vi "Read_CSV_Files_9234x2.vi"() -> ()   [LabVIEW 2022 SP3]
uses:
  <vilib>/express/express analysis/Spectral/Block/exnSpectralBlock spectral measurements peak poly.vi
  <vilib>/express/express analysis/Spectral/Block/exnSpectralBlock spectral measurements peak DDT.vi
  <vilib>/ErrorRing/Error Ring.xnode
  <vilib>/express/express analysis/Spectral/XNode/ExpressSpectralMeasurementsBlockNode.xnode
panel:
  in  "Rechose":bool
  in  "Rescan":bool
  in  "Data Connect":bool
  in  "FFT export":bool
  out "選擇/總資料":string
  in  "Filenames":i32(listbox)
  out "error out":errorcluster
  out "Timedomain":dynamicdata(graph)
  out "FFT":dynamicdata(graph)
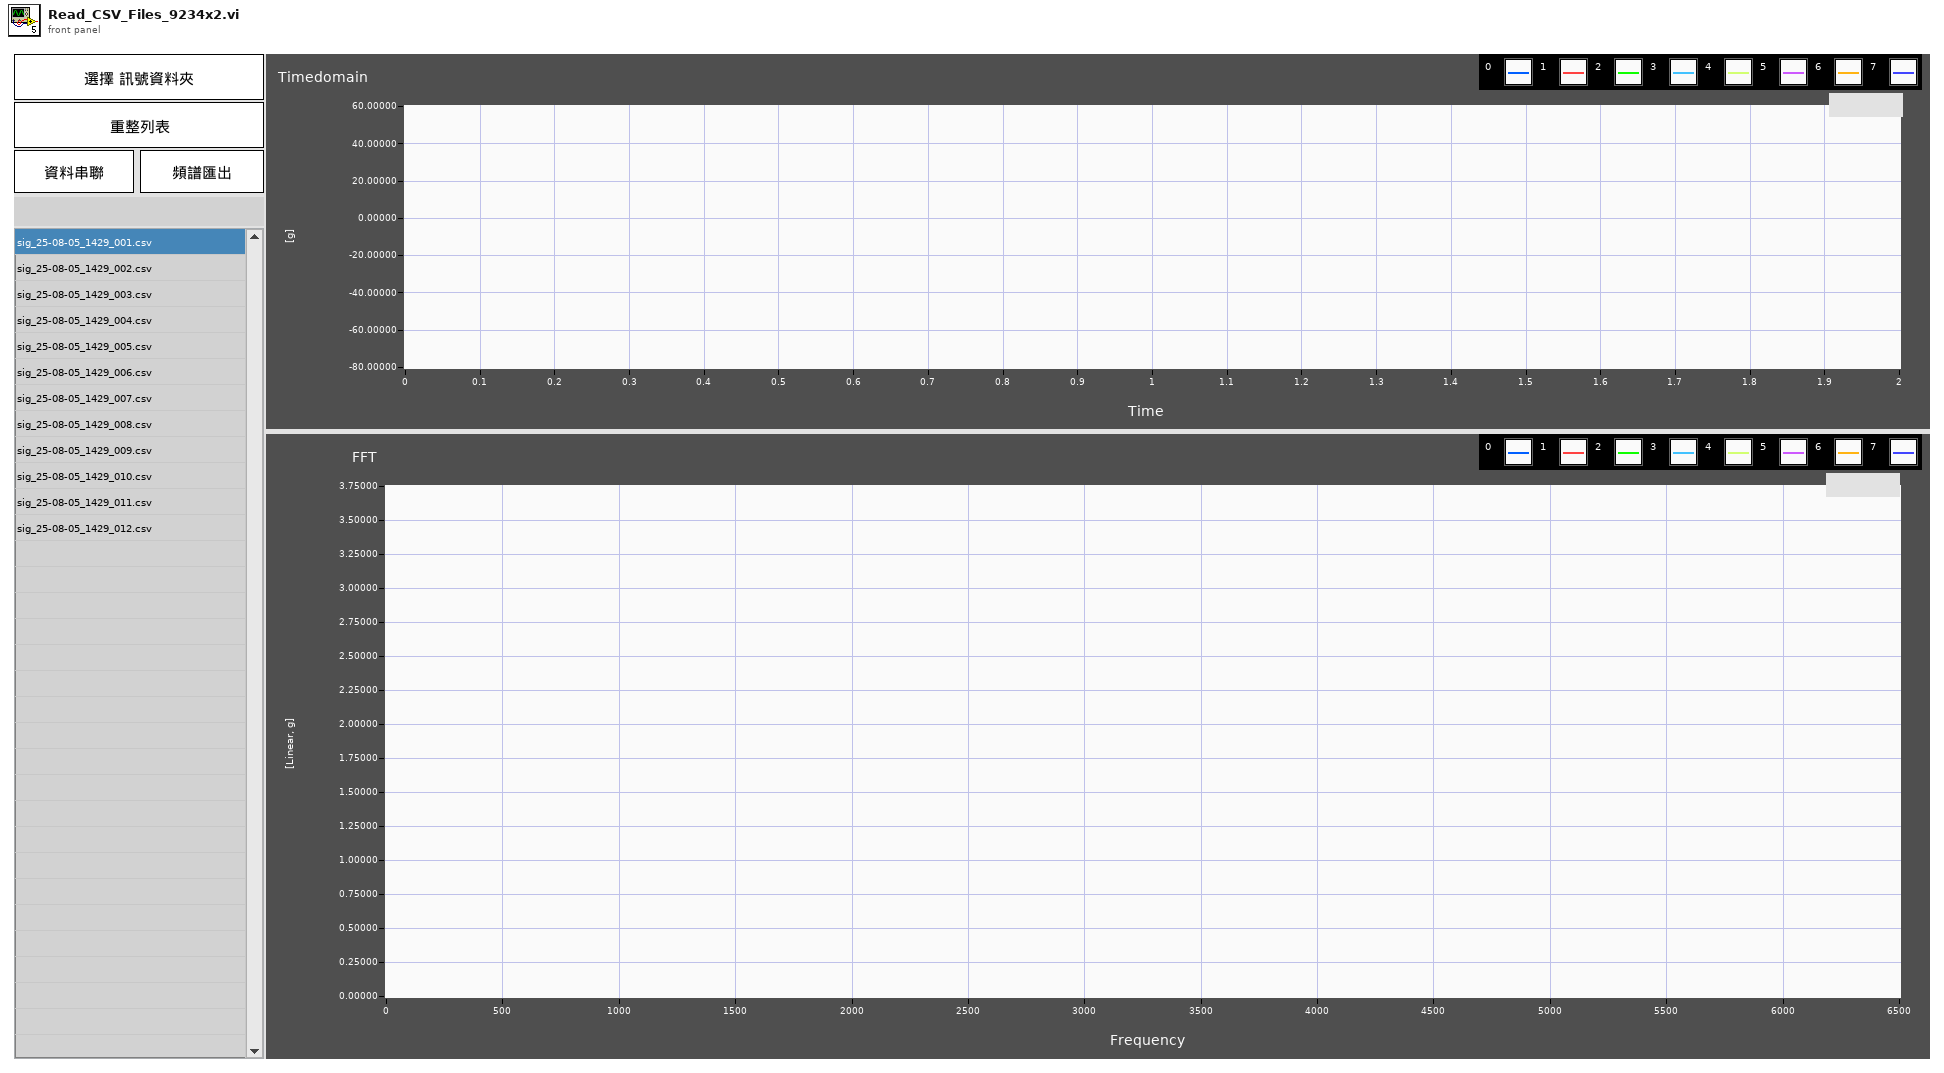
[diagram p1: front panel]
types:
  T1 = cluster{"averaging mode":u16, "weighting mode":u16, "number of averages":u32}
  T2 = cluster{"dB On (F)":bool, "unwrap phase (F)":bool, "convert to degree (F)":bool}
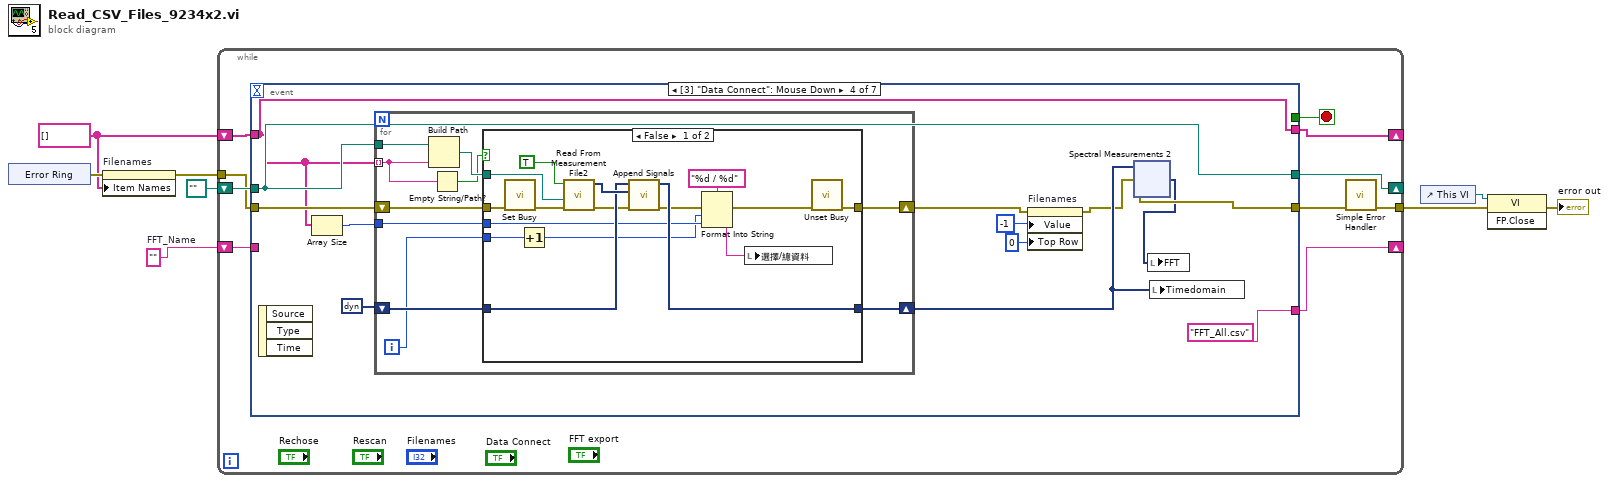
[diagram p0: block diagram]
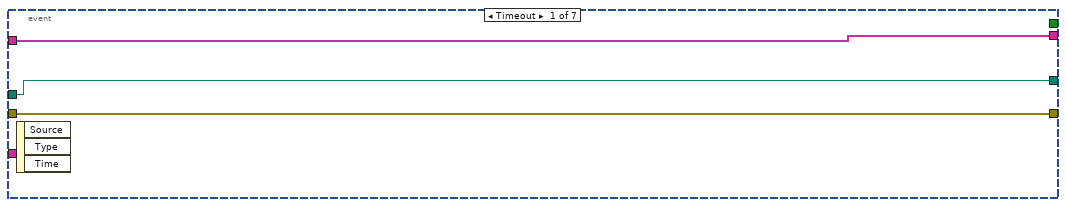
[diagram p2: hidden frame]
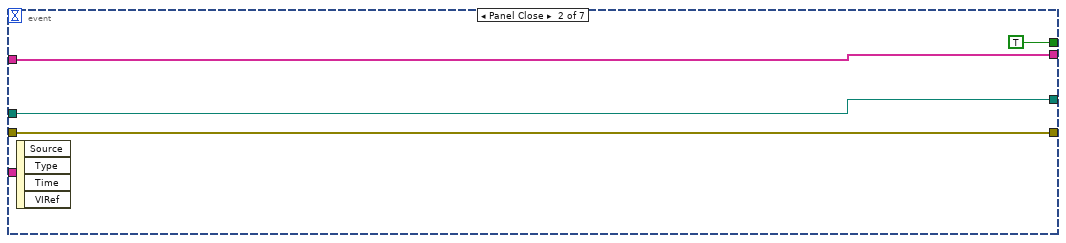
[diagram p3: hidden frame]
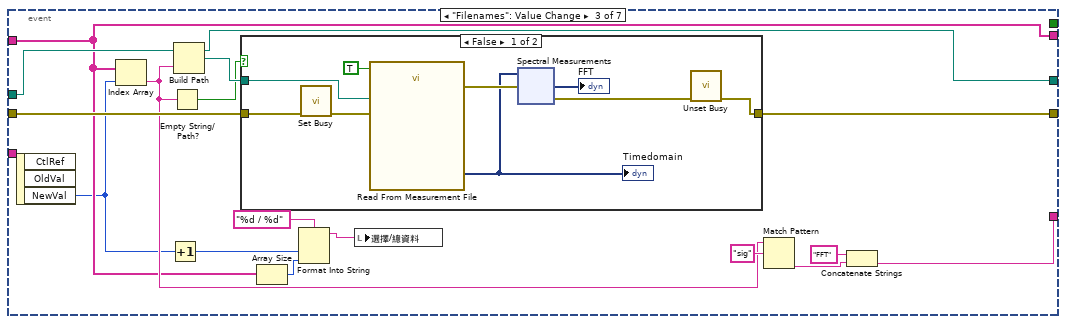
[diagram p4: hidden frame]
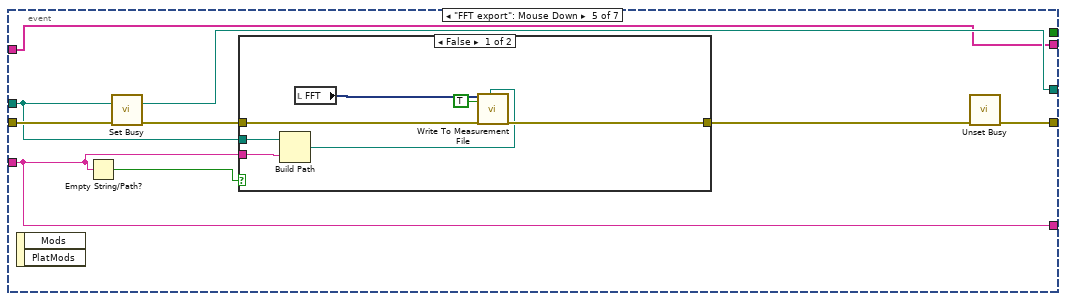
[diagram p7: hidden frame]
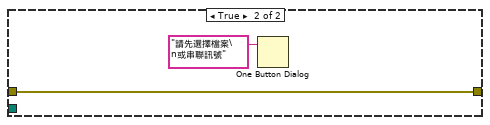
[diagram p8: hidden frame]
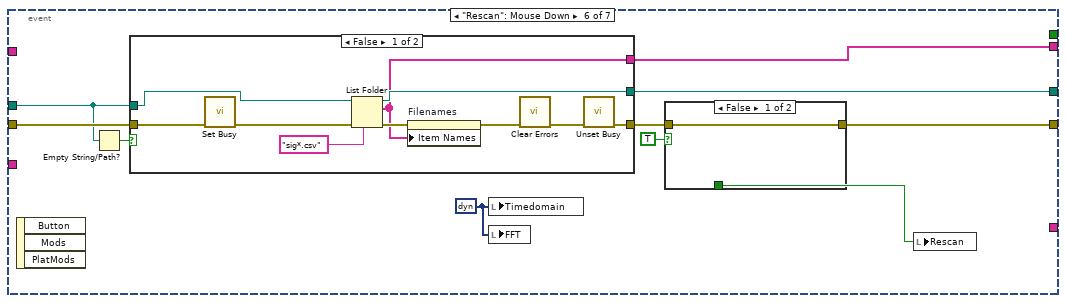
[diagram p9: hidden frame]
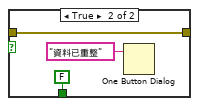
[diagram p10: hidden frame]
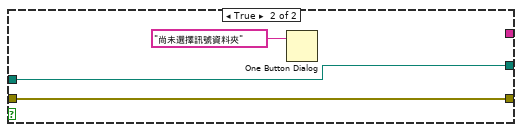
[diagram p11: hidden frame]
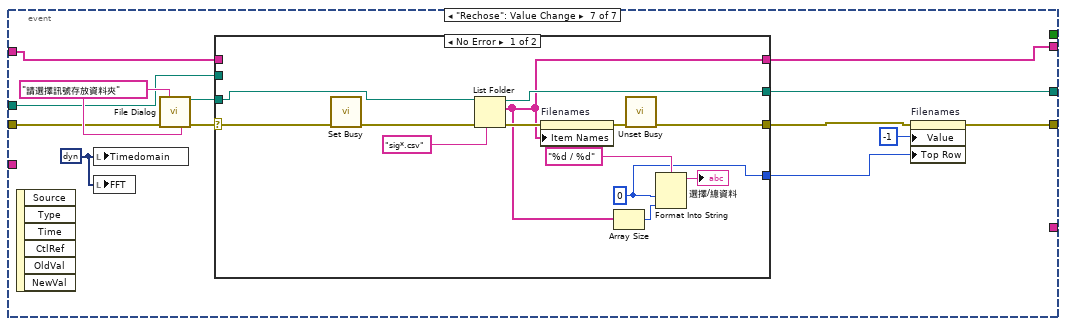
[diagram p12: hidden frame]
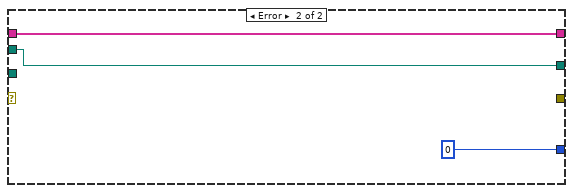
[diagram p13: hidden frame]
diagram:
  w1 = ""  # FFT_Name
  w2 = string[] [] ("filenames")
  n1 = xnode "Error Ring"() -> ("error out"=w4:errorcluster)
  n2 = property on="Filenames" class="LstBox (strict)"(error in=w4, "Item Names"=w2) -> (error out=w3:errorcluster)  [unwired: 1 in, 1 out]
  n3 = while {
    tunnel: [w14] -> w6
    shift-right: [w12] -> _
    shift-left: w2 -> [w16]
    shift-right: [w13] -> _
    shift-left: path "" ("path out") -> [w17]
    tunnel: w3 -> [w11]
    shift-right: [w10] -> _
    shift-left: w1 -> [w9]
    stop <- w18 stop-if-true
    n4 = event shown="[3] \"Data Connect\": Mouse Down" {
      selector: _ -> [_ _ _ _ _ _ _]
      dyn-events: _ -> [_ _ _ _ _ _ _]
      timeout: _ -> [_ _ _ _ _ _ _]
      tunnel: [w21 w24 w41 w72 w118 w132 w159] -> w15
      tunnel: [_ TRUE _ _ _ _ _] -> w18
      tunnel: w17 -> [w20 w23 w37 w73 w114 w136 w165]
      tunnel: w16 -> [w19 w22 w29 w67 w113 _ w164]
      tunnel: [w20 w23 w37 w73 w114 w139 w166] -> w13
      tunnel: [w19 w22 w29 w67 w113 w138 w167] -> w12
      tunnel: w11 -> [w21 w24 w38 w74 w120 w137 w162]
      tunnel: [_ _ w32 "FFT_All.csv" w115 _ _] -> w10
      tunnel: w9 -> [_ _ _ _ w115 _ _]
      event Timeout {
        n5 = event-data() -> ()  [unwired: 1 in, 3 out]
      }
      event Panel Close {
        n6 = event-data() -> ()  [unwired: 1 in, 4 out]
      }
      event "Filenames": Value Change {
        n7 = event-data() -> ("NewVal"=w28:i32)  [unwired: 1 in, 2 out]
        n8 = Index Array(array=w29, index=w28) -> (element=w33:string)
        n9 = Increment(x=w28) -> (x+1=w26:i32)
        n10 = Empty String/Path?(string/path=w33) -> (empty?=w39:bool)
        n11 = Build Path(base path=w37, name or relative path=w33) -> (appended path=w40:path)
        n12 = case shown="False" w39 {
          tunnel: [w47 w61] -> w41
          tunnel: w40 -> [w50 _]
          tunnel: w38 -> [w46 w61]
          frame False {
            n13 = call <vilib>:"Set Busy.vi"("error in (no error)"=w46) -> ("error out"=w48:errorcluster)  [unwired: 9 in, 1 out]
            n14 = call "Read From Measurement File"("error in (no error)"=w48, "Filename"=w50, "Reset"=TRUE) -> ("error out"=w45:errorcluster, "Signals"=w42:dynamicdata)  [unwired: 3 in, 4 out]
            "Timedomain" <- w42
            n15 = xnode ("Spectral Measurements")("Signals"=w42, "error in (no error)"=w45) -> ("FFT - (Peak)"=→"FFT":dynamicdata, "error out"=w44:errorcluster)  [unwired: 1 out]
            n16 = call <vilib>:"Unset Busy.vi"("error in (no error)"=w44) -> ("error out"=w47:errorcluster)  [unwired: 10 in]
          }
          frame True {
          }
        }
        n17 = Array Size(array=w29) -> (size(s)=w30:i32)
        n18 = Format Into String(format string="%d / %d", w26, w30) -> (resulting string=w27:string)  [unwired: 2 in, 1 out]
        n19 = local write "選擇/總資料"(w27) -> ()
        n20 = Match Pattern(string=w33, regular expression="sig") -> (after substring=w35:string)  [unwired: 1 in, 3 out]
        n21 = Concatenate Strings("FFT" ("string"), w35) -> (w32:string)
      }
      event "Data Connect": Mouse Down {
        n22 = event-data() -> ()  [unwired: 1 in, 3 out]
        n23 = Array Size(array=w67) -> (size(s)=w68:i32)
        n24 = for {
          tunnel: w73 -> [w89]
          tunnel: w67 -> [w92] mode=indexing
          shift-right: [w94] -> w65
          shift-left: w74 -> [w90]
          shift-right: [w87] -> w71
          shift-left: dynamicdata [] ("Signals") -> [w88]
          tunnel: w68 -> [w86]
          i -> [w85]
          n25 = Build Path(base path=w89, name or relative path=w92) -> (appended path=w93:path)
          n26 = Empty String/Path?(string/path=w92) -> (empty?=w91:bool)
          n27 = case shown="False" w91 {
            tunnel: [w107 w112] -> w94
            tunnel: w93 -> [w110 _]
            tunnel: w90 -> [w106 w112]
            tunnel: w88 -> [w104 w111]
            tunnel: [w103 w111] -> w87
            tunnel: w86 -> [w97 _]
            tunnel: w85 -> [w96 _]
            frame False {
              n28 = call <vilib>:"Set Busy.vi"("error in (no error)"=w106) -> ("error out"=w108:errorcluster)  [unwired: 9 in, 1 out]
              n29 = Increment(x=w96) -> (x+1=w95:i32)
              n30 = call "Read From Measurement File2"("error in (no error)"=w108, "Filename"=w110, "Reset"=TRUE) -> ("error out"=w102:errorcluster, "Signals"=w105:dynamicdata)  [unwired: 3 in, 4 out]
              n31 = call "Append Signals"("error in (no error)"=w102, "Input Signal B"=w105, "Input Signal A"=w104) -> ("error out"=w99:errorcluster, "Appended Signals"=w103:dynamicdata)  [unwired: 7 in]
              n32 = Format Into String(format string="%d / %d", error in=w99, w95, w97) -> (resulting string=w101:string, error out=w98:errorcluster)  [unwired: 1 in]
              n33 = local write "選擇/總資料"(w101) -> ()
              n34 = call <vilib>:"Unset Busy.vi"("error in (no error)"=w98) -> ("error out"=w107:errorcluster)  [unwired: 10 in]
            }
            frame True {
            }
          }
        }
        n35 = property on="Filenames" class="LstBox (strict)"(error in=w65, "Value"=-1 ("Filenames"), "Top Row"=0) -> (error out=w64:errorcluster)  [unwired: 1 in, 1 out]
        n36 = xnode ("Spectral Measurements 2")("Signals"=w71, "error in (no error)"=w64) -> ("FFT - (Peak)"=w70:dynamicdata, "error out"=w72:errorcluster)  [unwired: 1 out]
        n37 = local write "FFT"(w70) -> ()
        n38 = local write "Timedomain"(w71) -> ()
      }
      event "FFT export": Mouse Down {
        n39 = event-data() -> ()  [unwired: 1 in, 2 out]
        n40 = Empty String/Path?(string/path=w115) -> (empty?=w116:bool)
        n41 = call <vilib>:"Set Busy.vi"("error in (no error)"=w120) -> ("error out"=w119:errorcluster)  [unwired: 9 in, 1 out]
        n42 = case shown="False" w116 {
          tunnel: w119 -> [w126 w128]
          tunnel: [w125 w128] -> w117
          tunnel: w114 -> [w124 _]
          tunnel: w115 -> [w123 _]
          frame False {
            n43 = Build Path(base path=w124, name or relative path=w123) -> (appended path=w122:path)
            n44 = local read "FFT"() -> (w127:dynamicdata)
            n45 = call "Write To Measurement File"("Signals"=w127, "Reset"=TRUE, "error in (no error)"=w126, "Filename"=w122) -> ("error out"=w125:errorcluster)  [unwired: 13 in, 2 out]
          }
          frame True {
            n46 = One Button Dialog(message="請先選擇檔案\n或串聯訊號") -> ()  [unwired: 1 in, 1 out]
          }
        }
        n47 = call <vilib>:"Unset Busy.vi"("error in (no error)"=w117) -> ("error out"=w118:errorcluster)  [unwired: 10 in]
      }
      event "Rescan": Mouse Down {
        w134 = dynamicdata [] ("Timedomain")
        n48 = event-data() -> ()  [unwired: 1 in, 3 out]
        n49 = Empty String/Path?(string/path=w136) -> (empty?=w135:bool)
        n50 = case shown="False" w135 {
          tunnel: [w151 w154] -> w139
          tunnel: [w150 _] -> w138
          tunnel: [w148 w155] -> w131
          tunnel: w137 -> [w147 w155]
          tunnel: w136 -> [w144 w154]
          frame False {
            n51 = call <vilib>:"Set Busy.vi"("error in (no error)"=w147) -> ("error out"=w149:errorcluster)  [unwired: 9 in, 1 out]
            n52 = List Folder(path=w144, pattern="sig*.csv", error in=w149) -> (path out=w151:path, filenames=w150:string[], error out=w152:errorcluster)  [unwired: 1 in, 1 out]
            n53 = property on="Filenames" class="LstBox (strict)"(error in=w152, "Item Names"=w150) -> (error out=w146:errorcluster)  [unwired: 1 in, 1 out]
            n54 = call <vilib>:"Clear Errors.vi"("error in (no error)"=w146) -> ("error out"=w145:errorcluster)  [unwired: 5 in, 1 out]
            n55 = call <vilib>:"Unset Busy.vi"("error in (no error)"=w145) -> ("error out"=w148:errorcluster)  [unwired: 10 in]
          }
          frame True {
            n56 = One Button Dialog(message="尚未選擇訊號資料夾") -> ()  [unwired: 1 in, 1 out]
          }
        }
        n57 = local write "Timedomain"(w134) -> ()
        n58 = local write "FFT"(w134) -> ()
        n59 = case shown="False" TRUE {
          tunnel: [_ FALSE ("Rescan")] -> w133
          tunnel: [w140 w142] -> w132
          tunnel: w131 -> [w140 w142]
          frame False {
          }
          frame True {
            n60 = One Button Dialog(message="資料已重整") -> ()  [unwired: 1 in, 1 out]
          }
        }
        n61 = local write "Rescan"(w133) -> ()
      }
      event "Rechose": Value Change {
        w158 = dynamicdata [] ("Timedomain")
        w169 = "請選擇訊號存放資料夾" ("prompt")
        n62 = event-data() -> ()  [unwired: 1 in, 6 out]
        n63 = local write "Timedomain"(w158) -> ()
        n64 = local write "FFT"(w158) -> ()
        n65 = call "File Dialog"("prompt"=w169, "error in"=w162, "pattern label"=w169) -> ("selected path"=w168:path, "error out"=w163:errorcluster)  [unwired: 9 in, 2 out]
        n66 = case shown="No Error" w163 {
          selector: w163 -> [w175 _]
          tunnel: w168 -> [w180 _]
          tunnel: [w174 w184] -> w167
          tunnel: [w179 w185] -> w166
          tunnel: [w176 _] -> w160
          tunnel: w165 -> [_ w185]
          tunnel: w164 -> [_ w184]
          tunnel: [w171 0 ("Top Row")] -> w157
          frame No Error {
            w171 = 0 ("Top Row")
            n67 = call <vilib>:"Set Busy.vi"("error in (no error)"=w175) -> ("error out"=w177:errorcluster)  [unwired: 9 in, 1 out]
            n68 = List Folder(path=w180, pattern="sig*.csv", error in=w177) -> (path out=w179:path, filenames=w174:string[], error out=w181:errorcluster)  [unwired: 1 in, 1 out]
            n69 = property on="Filenames" class="LstBox (strict)"(error in=w181, "Item Names"=w174) -> (error out=w178:errorcluster)  [unwired: 1 in, 1 out]
            n70 = Array Size(array=w174) -> (size(s)=w172:i32)
            n71 = call <vilib>:"Unset Busy.vi"("error in (no error)"=w178) -> ("error out"=w176:errorcluster)  [unwired: 10 in]
            n72 = Format Into String(format string="%d / %d", w171, w172) -> (resulting string=→"選擇/總資料":string)  [unwired: 2 in, 1 out]
          }
          frame Error {
          }
        }
        n73 = property on="Filenames" class="LstBox (strict)"(error in=w160, "Value"=-1 ("Filenames"), "Top Row"=w157) -> (error out=w159:errorcluster)  [unwired: 1 in, 1 out]
      }
    }
    n74 = call <vilib>:"Simple Error Handler.vi"("error in (no error)"=w15) -> ("error out"=w14:errorcluster)  [unwired: 4 in, 4 out]
  }
  n75 = control-ref of="This VI"() -> (w7:refnum<vi>)
  n76 = invoke class="VI" method="FP.Close"(reference=w7, error in=w6) -> (error out=→"error out":errorcluster)  [unwired: 1 in, 2 out]
